vi "Initialize Axis.vi"(8 "error in (no error)":errorcluster, 10 "Number of Axis":i32, 11 "Joystick in":refnum<class "Joystick.lvclass">) -> (0 "error out":errorcluster, 3 "Joystick out":refnum<class "Joystick.lvclass">)   [LabVIEW 2014, in "Joystick.lvlib" / "Joystick.lvclass"]
uses:
  Joystick.lvclass
  Axis State.ctl
  Button State.ctl
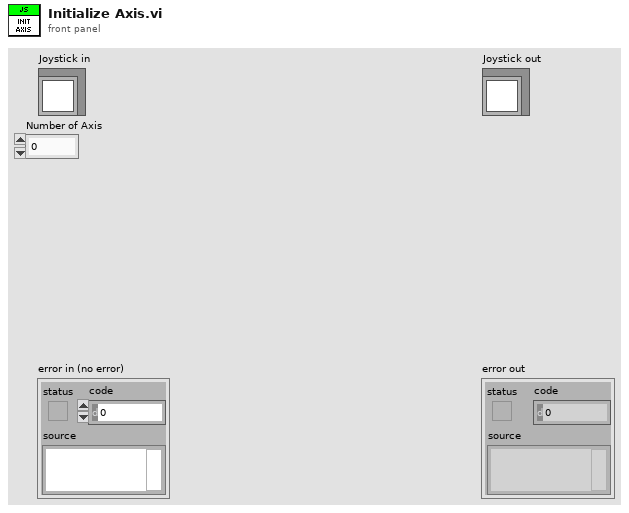
[diagram p1: front panel]
types:
  T1 = typedef "Joystick.lvlib/Joystick.lvclass/Axis State.ctl" = cluster{"Instance Name":string, "Deadband":dbl, "Value":dbl, "At Home":bool, "Postive Axis Button State":T2, "Negative Axis Button State":T2, "Home Axis Button State":T2}
  T2 = typedef "Joystick.lvlib/Joystick.lvclass/Button State.ctl" = cluster{"Pressed":bool, "Instance Name":string, "Toggled":bool, "Just Changed":bool}
  T3 = typedef "Joystick.lvlib/Joystick.lvclass/Joystick State.ctl" = cluster{"Buttons":T2[], "Axis":T1[]}
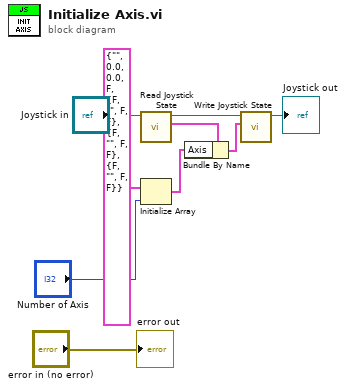
[diagram p0: block diagram]
diagram:
  n1 = call-dynamic "Read Joystick State.vi"("Joystick in"="Joystick in") -> ("Joystick State"=w5:T3, "Joystick out"=w8:refnum<class "Joystick.lvclass">)  [unwired: 8 in, 1 out]
  n2 = Initialize Array(T1 {"Instance Name"="", "Deadband"=0.0, "Value"=0.0, "At Home"=FALSE, "Postive Axis Button State"={"Pressed"=FALSE, "Instance Name"="", "Toggled"=FALSE, "Just Changed"=FALSE}, "Negative Axis Button State"={"Pressed"=FALSE, "Instance Name"="", "Toggled"=FALSE, "Just Changed"=FALSE}, "Home Axis Button State"={"Pressed"=FALSE, "Instance Name"="", "Toggled"=FALSE, "Just Changed"=FALSE}} ("Axis State"), "Number of Axis") -> (w1:T1[])
  n3 = Bundle By Name(cluster=w5, "Axis"=w1) -> (w2:T3)
  n4 = call-dynamic "Write Joystick State.vi"("Joystick State"=w2, "Joystick in"=w8) -> ("Joystick out"=→"Joystick out":refnum<class "Joystick.lvclass">)  [unwired: 8 in, 1 out]
  "error out" <- "error in (no error)"
